vi "OverlaySectorRoi.vi"(0 "Axis scaling Params":T1 {"Y high" format="%.2f"; "Y low" format="%.2f"; "X left" format="%.2f"; "X right" format="%.2f"}, 7 "Sector as Array":dbl[][](array[numeric]) format="%.2f", 9 "x coord":dbl[][](array[numeric]) format="%.2f", 11 "y coord":dbl[][](array[numeric]) format="%.2f", 12 "pixels in x":i16=250, 13 "pixels in y":i16=200) -> (4 "image overlay":dbl[][](array[numeric]) format="%.2f", 10 "x scaled":dbl[][](array[numeric]) format="%.2f", 15 "y scaled":dbl[][](array[numeric]) format="%.2f")   [LabVIEW 2022 SP3]
panel:
  out "Sector as data array":u8[][](graph)
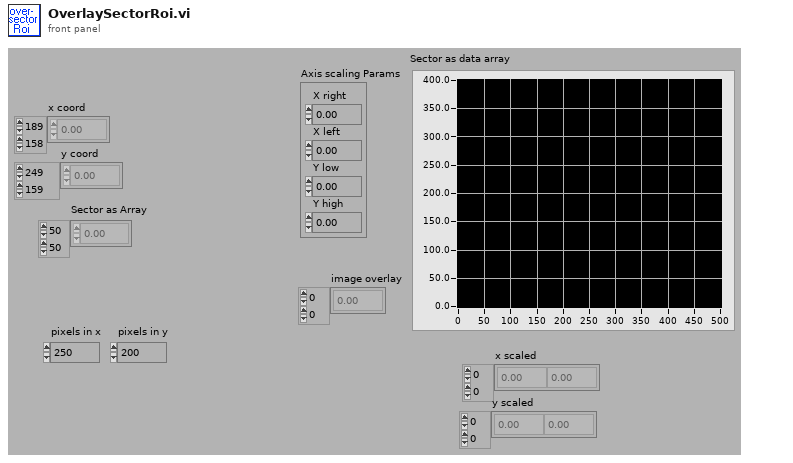
[diagram p1: front panel]
types:
  T1 = cluster{"X right":dbl, "X left":dbl, "Y low":dbl, "Y high":dbl}
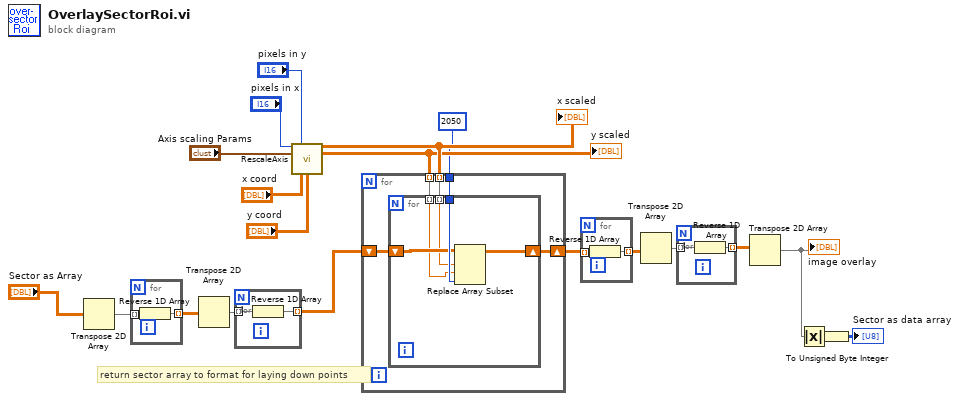
[diagram p0: block diagram]
diagram:
  # "return sector array to format for laying down points"
  n1 = Transpose 2D Array(2D array="Sector as Array") -> (transposed array=w3:dbl[][])
  n2 = for {
    tunnel: [w22] -> w18 mode=indexing
    tunnel: w3 -> [w21] mode=indexing
    n3 = Reverse 1D Array(array=w21) -> (reversed array=w22:dbl[])
  }
  n4 = Transpose 2D Array(2D array=w18) -> (transposed array=w19:dbl[][])
  n5 = for {
    tunnel: w19 -> [w23] mode=indexing
    tunnel: [w24] -> w7 mode=indexing
    n6 = Reverse 1D Array(array=w23) -> (reversed array=w24:dbl[])
  }
  n7 = call "RescaleAxis.vi"("pixels in x"="pixels in x", "pixels in y"="pixels in y", "Axis scaling Params"="Axis scaling Params", "x"="x coord", "y"="y coord") -> ("x scaled"=w17:dbl[][], "y scaled"=w16:dbl[][])  [unwired: 9 out]
  "x scaled" <- w17
  "y scaled" <- w16
  n8 = for {
    tunnel: w17 -> [w29] mode=indexing
    tunnel: w16 -> [w28] mode=indexing
    tunnel: i16 2050 -> [w27]
    shift-right: [w25] -> w12
    shift-left: w7 -> [w26]
    n9 = for {
      tunnel: w29 -> [w30] mode=indexing
      tunnel: w28 -> [w31] mode=indexing
      tunnel: w27 -> [w33]
      shift-right: [w34] -> w25
      shift-left: w26 -> [w32]
      n10 = Replace Array Subset(array=w32, new element=w33, index (row)=w30, index (col)=w31) -> (w34:dbl[][])
    }
  }
  n11 = for {
    tunnel: [w36] -> w14 mode=indexing
    tunnel: w12 -> [w35] mode=indexing
    n12 = Reverse 1D Array(array=w35) -> (reversed array=w36:dbl[])
  }
  n13 = Transpose 2D Array(2D array=w14) -> (transposed array=w15:dbl[][])
  n14 = for {
    tunnel: w15 -> [w37] mode=indexing
    tunnel: [w38] -> w2 mode=indexing
    n15 = Reverse 1D Array(array=w37) -> (reversed array=w38:dbl[])
  }
  n16 = Transpose 2D Array(2D array=w2) -> (transposed array=w1:dbl[][])
  "image overlay" <- w1
  n17 = Absolute Value(x=w1) -> (abs(x)=w9:dbl[][])
  n18 = To Unsigned Byte Integer(number=w9) -> (unsigned 8bit integer=→"Sector as data array":u8[][])
